vi "wd_addRecordInOneNode (WFM).vi"(6 "length":u64, 7 "waveform":waveform(dbl), 8 "error in (no error)":errorcluster, 9 "start":u64, 10 "datalog postion":i64, 11 "meta in":T1={"TargetFile"=path "", "StreamMode"=enum."File", "Append?"=FALSE, "ChunkSize"=0, "TimeColumnMode"=enum."Empty", "TimestampFormat"="", "AbsoluteTime?"=FALSE, "FileAttribute "={"Creator"="", "Title"="", "SheetName"=""}, "Column"=[], "FileRef"=refnum, "MemoryRef"=[], "RecordInfo"=[], " ChannelPreviousInfo"=[], "ChannelFirstRecord"=[], "PredefinedFormattedValueLength"=20, "DiskTemplate"={"XMLRef"=[refnum, refnum, refnum, refnum, refnum, refnum], "ZipPath"=path "", "MetaFile"={"Ref"=refnum, "NextRow"=0, "NextPosition"=0, "Block"=[]}, "TempFolder"=path ""}}) -> (0 "error out":errorcluster, 3 "meta out":T1={"TargetFile"=path "", "StreamMode"=enum."File", "Append?"=FALSE, "ChunkSize"=0, "TimeColumnMode"=enum."Empty", "TimestampFormat"="", "AbsoluteTime?"=FALSE, "FileAttribute "={"Creator"="", "Title"="", "SheetName"=""}, "Column"=[], "FileRef"=refnum, "MemoryRef"=[], "RecordInfo"=[], " ChannelPreviousInfo"=[], "ChannelFirstRecord"=[], "PredefinedFormattedValueLength"=20, "DiskTemplate"={"XMLRef"=[refnum, refnum, refnum, refnum, refnum, refnum], "ZipPath"=path "", "MetaFile"={"Ref"=refnum, "NextRow"=0, "NextPosition"=0, "Block"=[]}, "TempFolder"=path ""}}, 4 "waveform out":waveform(dbl))   [LabVIEW 2020, in "NI_ExcelFile.lvlib"]
uses:
  <vilib>/express/express shared/NI_ExcelFile/NI_ExcelFile.lvlib
  <vilib>/express/express shared/NI_ExcelFile/Ctrls/MainData.ctl
  <vilib>/express/express shared/NI_ExcelFile/Ctrls/StreamMode.ctl
  <vilib>/express/express shared/NI_ExcelFile/Ctrls/TimeColumnMode.ctl
  <vilib>/express/express shared/NI_ExcelFile/Ctrls/FileAttribute.ctl
  <vilib>/express/express shared/NI_ExcelFile/Ctrls/Columns.ctl
  <vilib>/express/express shared/NI_ExcelFile/Ctrls/ColumnInfo.ctl
  <vilib>/express/express shared/NI_ExcelFile/Ctrls/DataType.ctl
  <vilib>/express/express shared/NI_ExcelFile/Ctrls/wd_recordInfo.ctl
  <vilib>/express/express shared/NI_ExcelFile/Ctrls/disk_TemplateFile.ctl
  <vilib>/express/express shared/NI_ExcelFile/Ctrls/meta_file.ctl
  <vilib>/express/express shared/NI_ExcelFile/Ctrls/meta_Block.ctl
  <vilib>/express/express shared/NI_ExcelFile/Ctrls/meta_BlockType.ctl
  <vilib>/express/express shared/NI_ExcelFile/SubVIs/utilities_addTime.vi
  <vilib>/Waveform/WDTOps.llb/WDT Append Waveforms DBL.vi
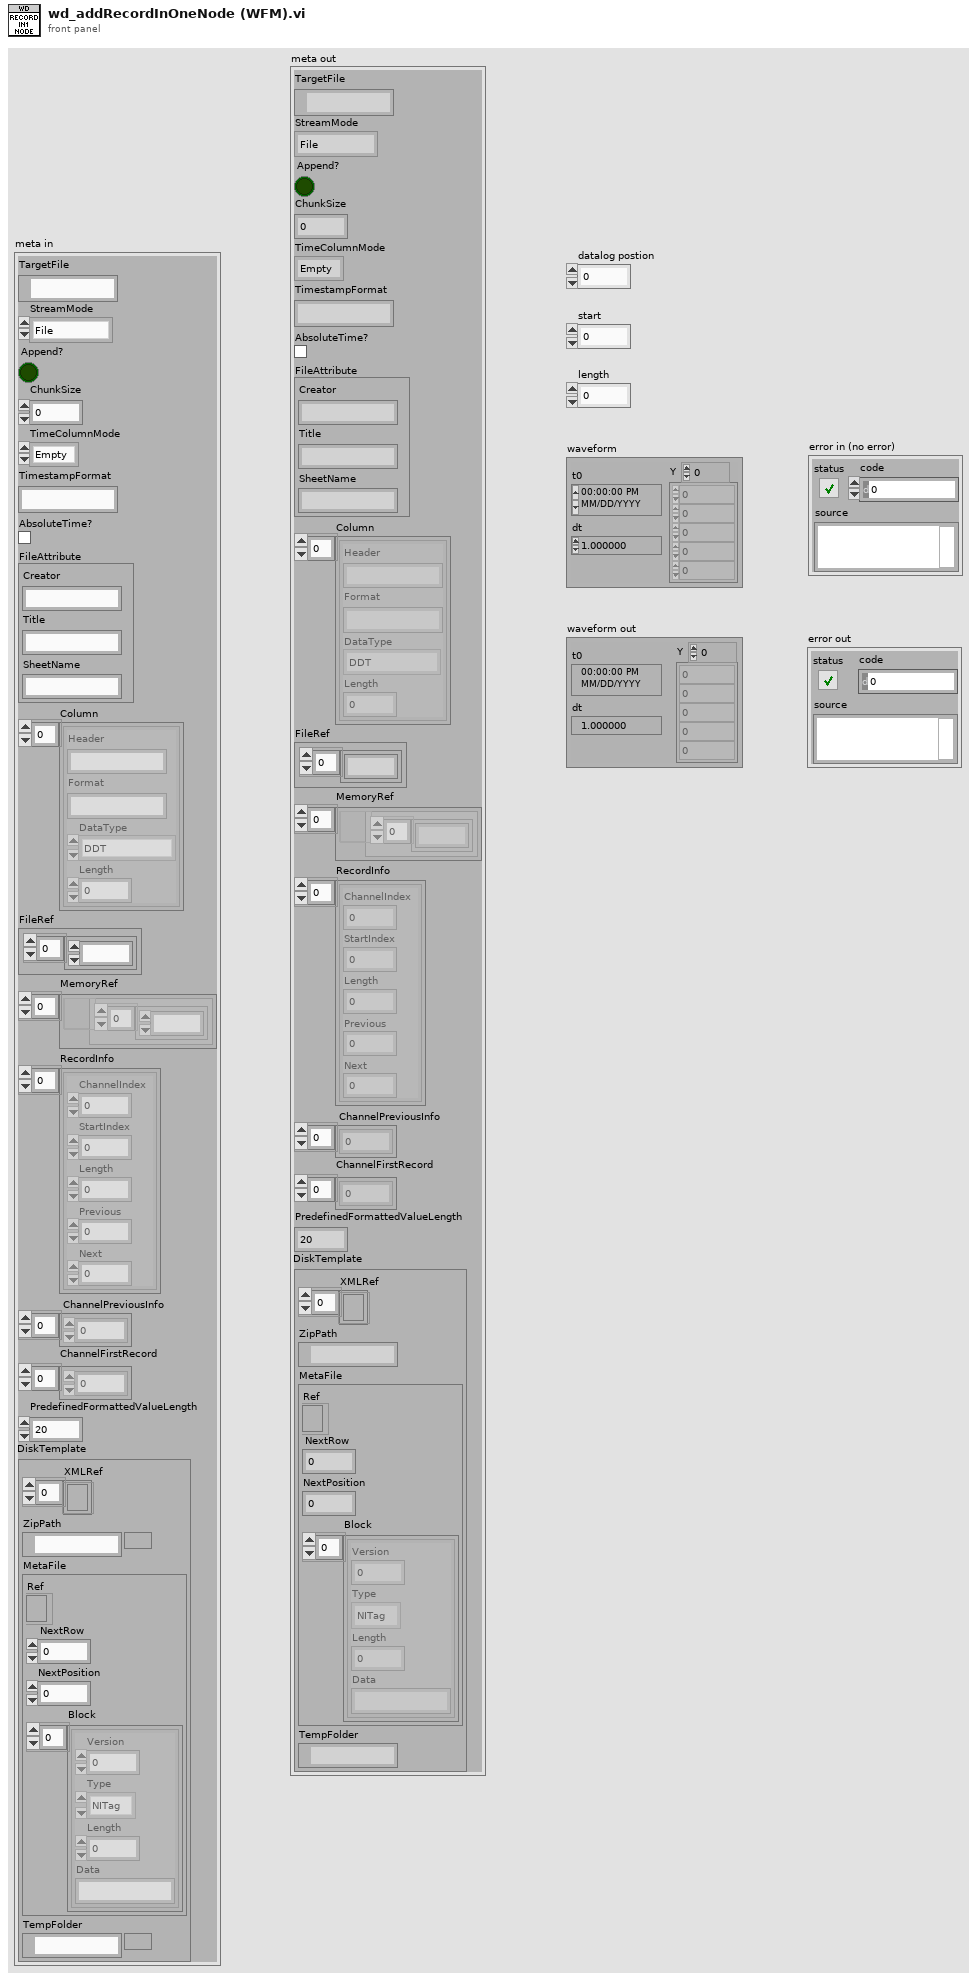
[diagram p1: front panel]
types:
  T1 = typedef "NI_ExcelFile.lvlib/MainData.ctl" = cluster{"TargetFile":path, "StreamMode":T2, "Append?":bool, "ChunkSize":u64, "TimeColumnMode":T3, "TimestampFormat":string, "AbsoluteTime?":bool, "FileAttribute ":T4, "Column":T5, "FileRef":refnum<k1>, "MemoryRef":refnum<data-value>[], "RecordInfo":T8[], " ChannelPreviousInfo":u32[], "ChannelFirstRecord":u32[], "PredefinedFormattedValueLength":i64, "DiskTemplate":T9}
  T2 = typedef "NI_ExcelFile.lvlib/StreamMode.ctl" = enum16{"File", "Memory"}
  T3 = typedef "NI_ExcelFile.lvlib/TimeColumnMode.ctl" = enum16{"Empty", "OnePerCh", "One"}
  T4 = typedef "NI_ExcelFile.lvlib/FileAttribute.ctl" = cluster{"Creator":string, "Title":string, "SheetName":string}
  T5 = typedef "NI_ExcelFile.lvlib/Columns.ctl" = T6[]
  T6 = typedef "NI_ExcelFile.lvlib/ColumnInfo.ctl" = cluster{"Header":string, "Format":string, "DataType":T7, "Length":u64}
  T7 = typedef "NI_ExcelFile.lvlib/DataType.ctl" = enum16{"DDT", "WFM", "Array of STR", "Array of DBL", "Array of I8", "Array of I16", "Array of I32", "Array of I64", "Array of SGL", "Array of U8", "Array of U16", "Array of U32", "Array of U64", "Array of Time"}
  T8 = typedef "NI_ExcelFile.lvlib/wd_recordInfo.ctl" = cluster{"ChannelIndex":u32, "StartIndex":u64, "Length":u64, "Previous":i32, "Next":i32}
  T9 = typedef "NI_ExcelFile.lvlib/disk_TemplateFile.ctl" = cluster{"XMLRef":refnum<file>[], "ZipPath":path, "MetaFile":T10, "TempFolder":path}
  T10 = typedef "NI_ExcelFile.lvlib/meta_file.ctl" = cluster{"Ref":refnum<file>, "NextRow":i32, "NextPosition":i64, "Block":T11[]}
  T11 = typedef "NI_ExcelFile.lvlib/meta_Block.ctl" = cluster{"Version":u16, "Type":T12, "Length":i32, "Data":string}
  T12 = typedef "NI_ExcelFile.lvlib/meta_BlockType.ctl" = enum16{"NITag", "File", "Column"}
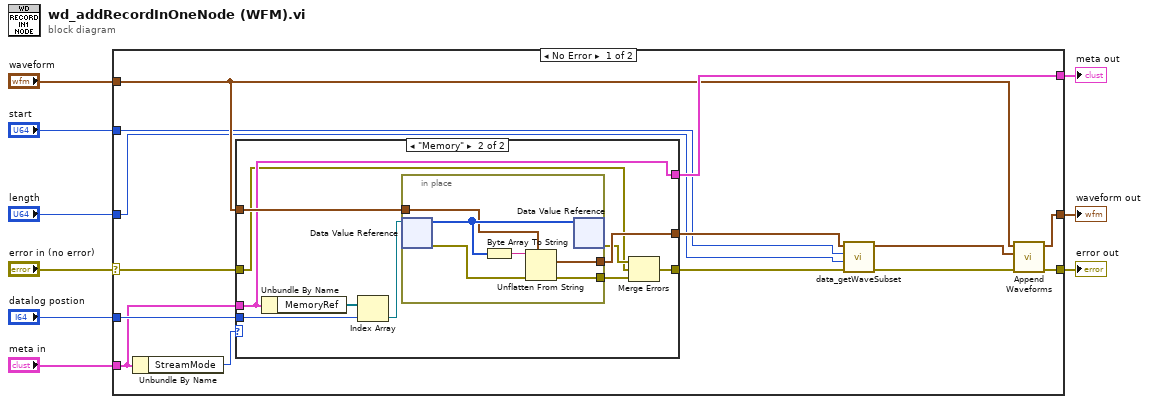
[diagram p0: block diagram]
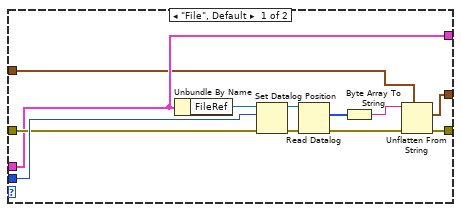
[diagram p2: hidden frame]
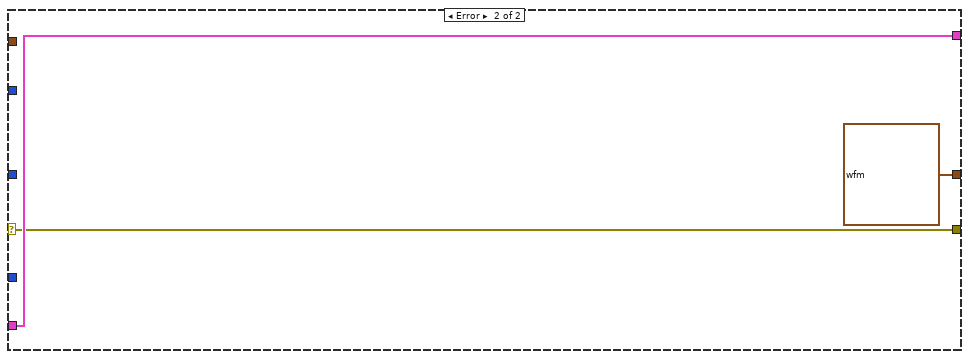
[diagram p3: hidden frame]
diagram:
  n1 = case shown="No Error" "error in (no error)" {
    selector: "error in (no error)" -> [w19 w53]
    tunnel: "datalog postion" -> [w23 _]
    tunnel: [w13 waveform(dbl) {"t0"=timestamp(0 s since 1904-01-01), "dt"=1.0, "Y"=[]} ("waveform out")] -> w1
    tunnel: "meta in" -> [w22 w54]
    tunnel: [w20 w54] -> w7
    tunnel: [w12 w53] -> w6
    tunnel: "waveform" -> [w14 _]
    tunnel: "start" -> [w10 _]
    tunnel: "length" -> [w11 _]
    frame No Error {
      n2 = Unbundle By Name(w22) -> ("StreamMode"=w21:T2)
      n3 = case shown="\"Memory\"" w21 {
        tunnel: w22 -> [w27 w41]
        tunnel: w19 -> [w29 w38]
        tunnel: w23 -> [w31 w42]
        tunnel: [w27 w41] -> w20
        tunnel: w14 -> [w26 w44]
        tunnel: [w25 w40] -> w16
        tunnel: [w24 w36] -> w17
        frame "File", Default {
          n4 = Unbundle By Name(w27) -> ("FileRef"=w30:refnum<k1>)
          n5 = Set Datalog Position(4:w29, 6:w31, 7:w30) -> (0:w35:errorcluster, 3:w32:refnum<k1>)  [unwired: 1 in]
          n6 = Read Datalog(4:w35, 7:w32) -> (0:w28:errorcluster, 2:w33:u8[])  [unwired: 1 in, 1 out]
          n7 = Byte Array To String(unsigned byte array=w33) -> (string=w34:string)
          n8 = Unflatten From String(type=w26, binary string=w34, error in (no error)=w28) -> (value=w25:waveform(dbl), error out=w24:errorcluster)  [unwired: 2 in, 1 out]
        }
        frame "Memory" {
          n9 = Unbundle By Name(w41) -> ("MemoryRef"=w43:refnum<data-value>[])
          n10 = Index Array(array=w43, index=w42) -> (element=w45:refnum<data-value>)
          n11 = in-place {
            in-place-border: w44 -> [w48]
            in-place-border: [w47] -> w40
            in-place-border: [w46] -> w37
            n12 = in-place-dvr #1(w45) -> (w50:u8[], w49:errorcluster)
            n13 = Byte Array To String(unsigned byte array=w50) -> (string=w51:string)
            n14 = Unflatten From String(type=w48, binary string=w51, error in (no error)=w49) -> (value=w47:waveform(dbl), error out=w46:errorcluster)  [unwired: 2 in, 1 out]
            n15 = in-place-dvr #1(w50) -> (w39:errorcluster)  [unwired: 1 out]
          }
          n16 = Merge Errors(w39, w38, w37) -> (w36:errorcluster)
        }
      }
      n17 = call <vilib>:"data_getWaveSubset.vi"("error in (no error)"=w17, "length"=w11, "index"=w10, "Waveform"=w16) -> ("error out"=w18:errorcluster, "Waveform out"=w15:waveform(dbl))  [unwired: 6 in]
      n18 = call-poly <vilib>:"Append Waveforms.vi"("error in (no error)"=w18, "waveform B"=w15, "waveform A"=w14) -> ("error out"=w12:errorcluster, "waveform out"=w13:waveform(dbl))  [unwired: 7 in]
    }
    frame Error {
    }
  }
  "meta out" <- w7
  "error out" <- w6
  "waveform out" <- w1
